vi "2photocell+ledcontrol+sum_cal4.vi"() -> ()   [LabVIEW 2016]
uses:
  <vilib>/LabVIEW Interface for Arduino/LabVIEW Interface for Arduino.lvlib
  <vilib>/ptbypt/NI_PtbyPt.lvlib
panel:
  in  "stop":bool
  in  "Tab Control":enum32{"Page 1", "Page 2", "Page 3"}(tab)
  out "Voltage 1":dbl(knob) scale=0.0..5.0
  out "alarm":bool
  out "LUX":string="Error"
  out "Filtered x 1":dbl format="%0.2f"
  in  "br_coef":dbl
  in  "thrs low":i32=1
  in  "thrs high":i32=4
  in  "q":dbl
  in  "p":dbl
  in  "k":dbl
  in  "thrs up":dbl
  in  "thrs down":dbl
  in  "Slide 3":dbl(slide) min=0.0 max=255.0 scale=0.0..255.0
  in  "Slide 2":dbl(slide) min=0.0 max=255.0 scale=0.0..255.0
  in  "Slide":dbl(slide) min=0.0 max=255.0 scale=0.0..255.0
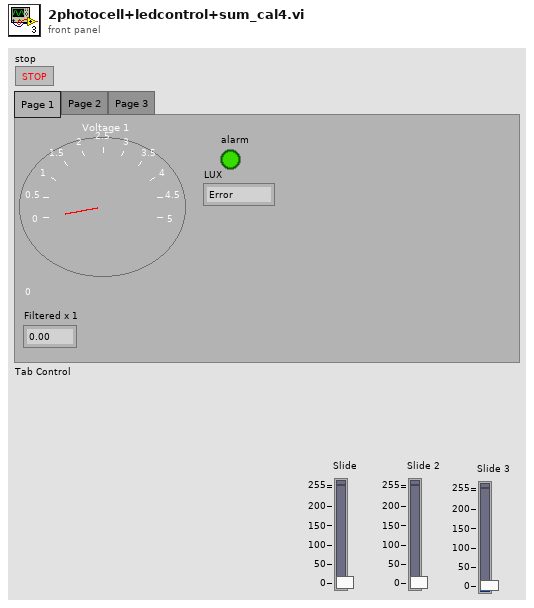
[diagram p1: front panel]
types:
  T1 = typedef "LabVIEW Interface for Arduino.lvlib/Arduino Resource.ctl" = cluster{"VISA resource":refnum<visa-resource-name>, "Board Type":T2, "Connection Type":enum8{"USB / Serial"}, "Bytes Per Packet (15)":u8}
  T2 = typedef "LabVIEW Interface for Arduino.lvlib/Board Type.ctl" = enum16{"Uno", "Dimuelanove w/Atmega 328", "Mega 2560"}
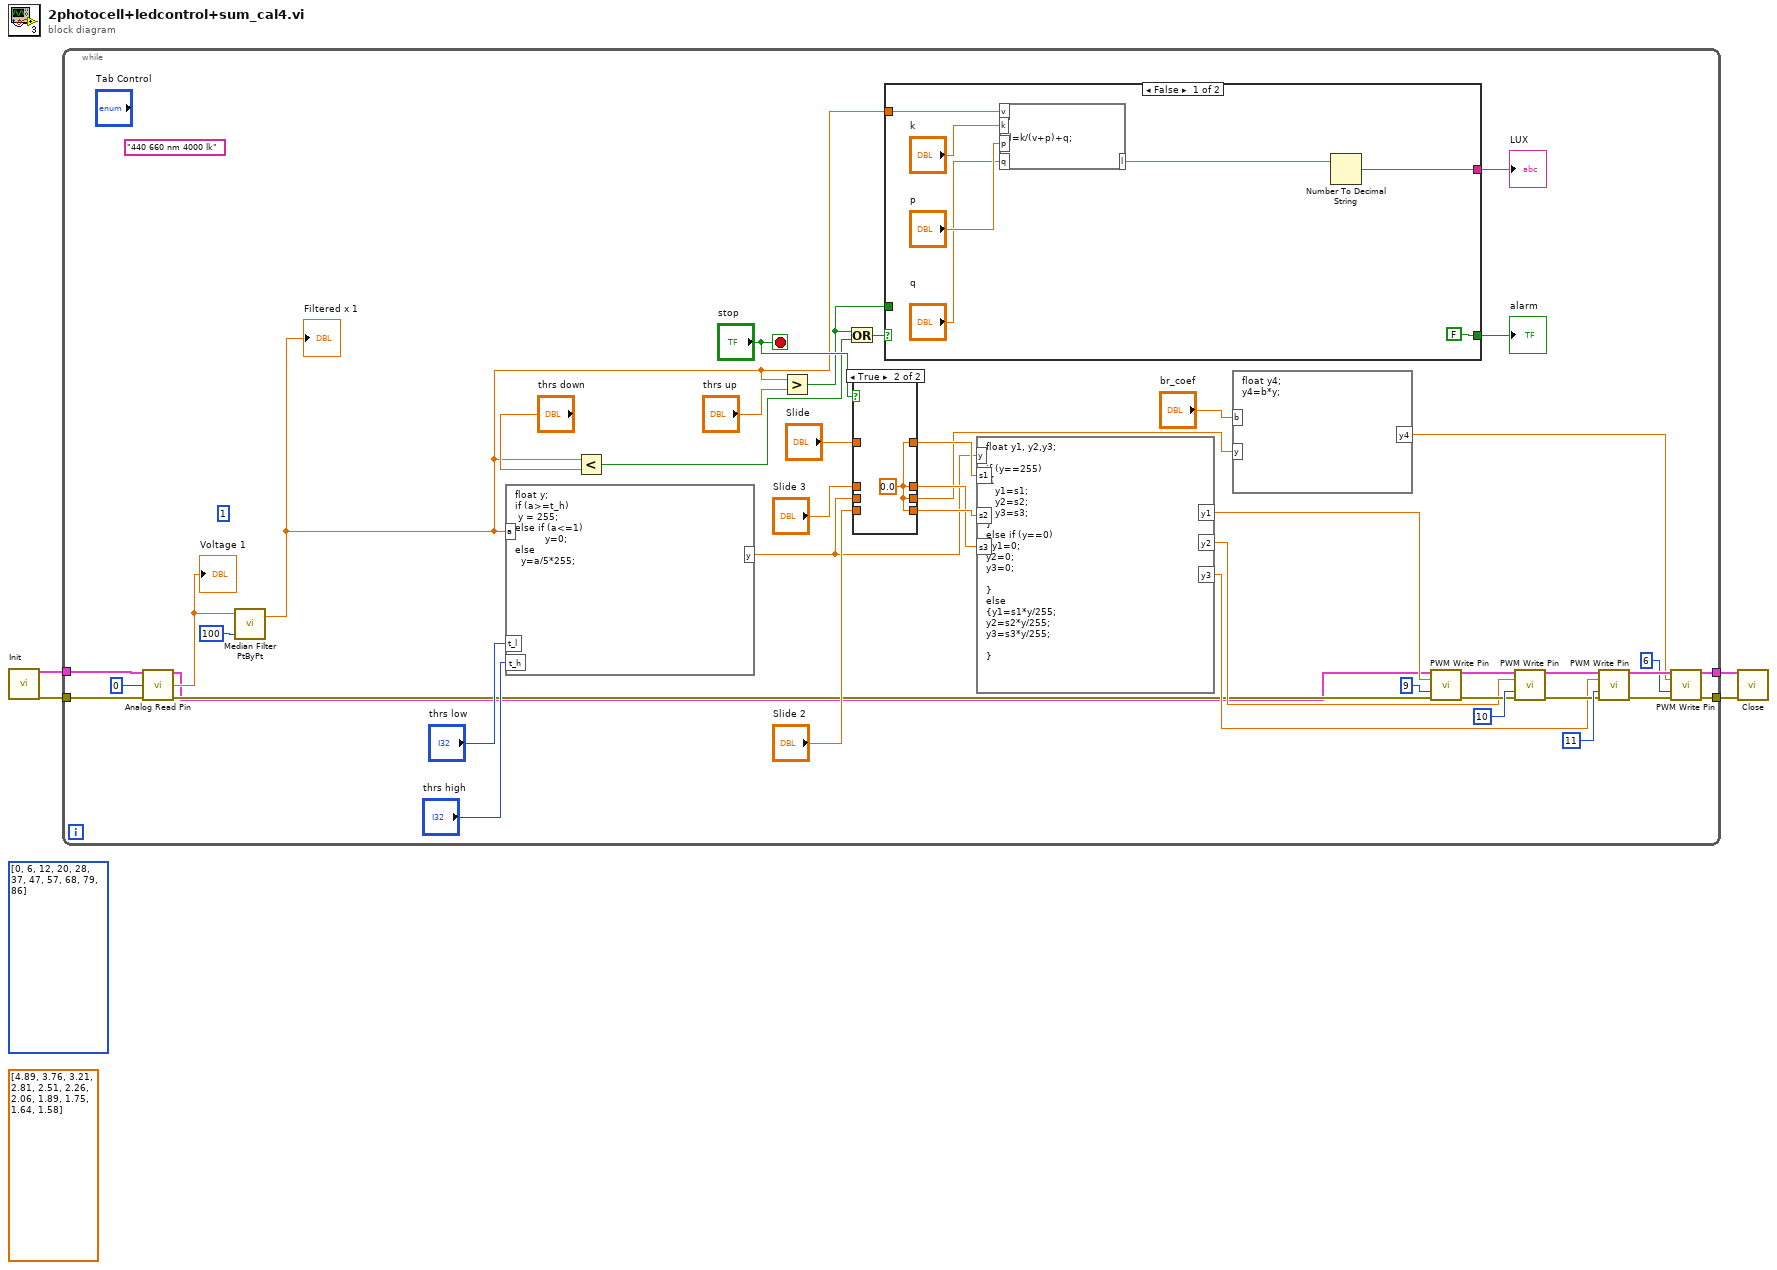
[diagram p0: block diagram]
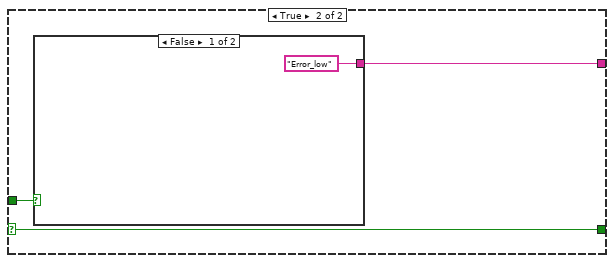
[diagram p2: hidden frame]
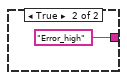
[diagram p3: hidden frame]
diagram:
  (unwired) dbl[] [4.89, 3.76, 3.21, 2.81, 2.51, 2.26, 2.06, 1.89, 1.75, 1.64, 1.58]
  (unwired) i32[] [0, 6, 12, 20, 28, 37, 47, 57, 68, 79, 86]
  n1 = call <vilib>:"Init.vi"() -> ("Arduino Resource"=w3:T1, "error out"=w4:errorcluster)  [unwired: 18 in]
  n2 = while {
    tunnel: w4 -> [w46]
    tunnel: w3 -> [w8]
    tunnel: [w23] -> w2
    tunnel: [w22] -> w1
    stop <- "stop" stop-if-true
    (unwired) u8 1 ("Analog Input Pin (0)")
    (unwired) "440 660 nm 4000 lk"
    n3 = call <vilib>:"Analog Read Pin.vi"("Arduino Resource"=w8, "Analog Input Pin (0)"=u8 0, "error in"=w46) -> ("Arduino Resource"=w6:T1, "Voltage"=w44:dbl, "error out"=w7:errorcluster)  [unwired: 10 in]
    "Voltage 1" <- w44
    n4 = call <vilib>:"Median Filter PtByPt.vi"("rank"=100, "x"=w44) -> ("Filtered x"=w5:dbl)  [unwired: 2 in, 1 out]
    "Filtered x 1" <- w5
    n5 = formula code="float y;\nif (a>=t_h)\n y = 255;\nelse if (a<=1)\n          y=0;\nelse\n  y=a/5*255;"("a"=w5, "t_l"="thrs low", "t_h"="thrs high") -> ("y"=w19:dbl)
    n6 = Less?(x=w5, y="thrs down") -> (x < y?=w13:bool)
    n7 = Greater?(x=w5, y="thrs up") -> (0:w9:bool)
    n8 = Or(x=w9, y=w13) -> (x .or. y?=w12:bool)
    n9 = case shown="True" "stop" {
      tunnel: "Slide 2" -> [w63 _]
      tunnel: [w63 w64] -> w29
      tunnel: "Slide 3" -> [w62 _]
      tunnel: [w62 w64] -> w28
      tunnel: "Slide" -> [w61 _]
      tunnel: [w61 w64] -> w30
      tunnel: w19 -> [w60 _]
      tunnel: [w60 w64] -> w17
      frame False {
      }
      frame True {
        w64 = 0.0 ("Slide 2")
      }
    }
    n10 = case shown="False" w12 {
      selector: w12 -> [_ w57]
      tunnel: [FALSE w57] -> w11
      tunnel: w5 -> [w53 _]
      tunnel: [w51 w55] -> w10
      tunnel: w9 -> [_ w56]
      frame False {
        n11 = formula code="l=k/(v+p)+q;"("v"=w53, "k"="k", "p"="p", "q"="q") -> ("l"=w52:dbl)
        n12 = Number To Decimal String(number=w52) -> (decimal integer string=w51:string)  [unwired: 1 in]
      }
      frame True {
        n13 = case shown="False" w56 {
          tunnel: ["Error_low" "Error_high"] -> w55
          frame False {
          }
          frame True {
          }
        }
      }
    }
    "alarm" <- w11
    "LUX" <- w10
    n14 = formula code="float y1, y2,y3;\n\nif (y==255)\n {\n   y1=s1;\n   y2=s2;\n   y3=s3;\n}\nelse if (y==0)\n{y1=0;\ny2=0;\ny3=0;\n\n}\nelse \n{y1=s1*y/255;\ny2=s2*y/255;\ny3=s3*y/255;\n\n}"("s1"=w30, "s2"=w29, "s3"=w28, "y"=w19) -> ("y1"=w27:dbl, "y2"=w26:dbl, "y3"=w25:dbl)
    n15 = formula code="float y4;\ny4=b*y;"("b"="br_coef", "y"=w17) -> ("y4"=w16:dbl)
    n16 = call <vilib>:"PWM Write Pin.vi"("Arduino Resource"=w6, "Duty Cycle (0 - 255)"=w27, "PWM Pin (3)"=u8 9, "error in"=w7) -> ("Arduino Resource"=w36:T1, "error out"=w32:errorcluster)  [unwired: 10 in]
    n17 = call <vilib>:"PWM Write Pin.vi"("Arduino Resource"=w36, "Duty Cycle (0 - 255)"=w26, "PWM Pin (3)"=u8 10, "error in"=w32) -> ("Arduino Resource"=w35:T1, "error out"=w31:errorcluster)  [unwired: 10 in]
    n18 = call <vilib>:"PWM Write Pin.vi"("Arduino Resource"=w35, "Duty Cycle (0 - 255)"=w25, "PWM Pin (3)"=u8 11, "error in"=w31) -> ("Arduino Resource"=w24:T1, "error out"=w21:errorcluster)  [unwired: 10 in]
    n19 = call <vilib>:"PWM Write Pin.vi"("Arduino Resource"=w24, "Duty Cycle (0 - 255)"=w16, "PWM Pin (3)"=u8 6, "error in"=w21) -> ("Arduino Resource"=w23:T1, "error out"=w22:errorcluster)  [unwired: 10 in]
  }
  n20 = call <vilib>:"Close.vi"("Arduino Resource"=w2, "error in"=w1) -> ()  [unwired: 13 in, 1 out]
